vi "TrajectoryDashWrite.vi"(8 "error in (no error)":errorcluster) -> (0 "error out":errorcluster)   [LabVIEW 2023]
uses:
  <vilib>/Rock Robotics/Network Tables/NT Write Boolean.vi
  <vilib>/Rock Robotics/Network Tables/NT Write Numeric Array.vi
  TrajectoryGlobals.vi
  <vilib>/Rock Robotics/Network Tables/NT Write Number.vi
  <vilib>/Rock Robotics/WPI/ThirdParty/JAS_Junk/TrajLib/Trajectory_Library.lvlib
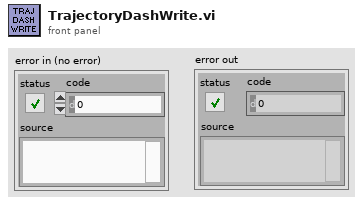
[diagram p1: front panel]
types:
  T1 = typedef "Trajectory_Library.lvlib/POSE2D.ctl" = cluster{"TRANSLATION":T2, "ROTATION":T3}
  T2 = typedef "Trajectory_Library.lvlib/TRANSLATION2D.ctl" = cluster{"X":dbl, "Y":dbl}
  T3 = typedef "Trajectory_Library.lvlib/ROTATION2D.ctl" = cluster{"VALUE":dbl, "COS":dbl, "SIN":dbl}
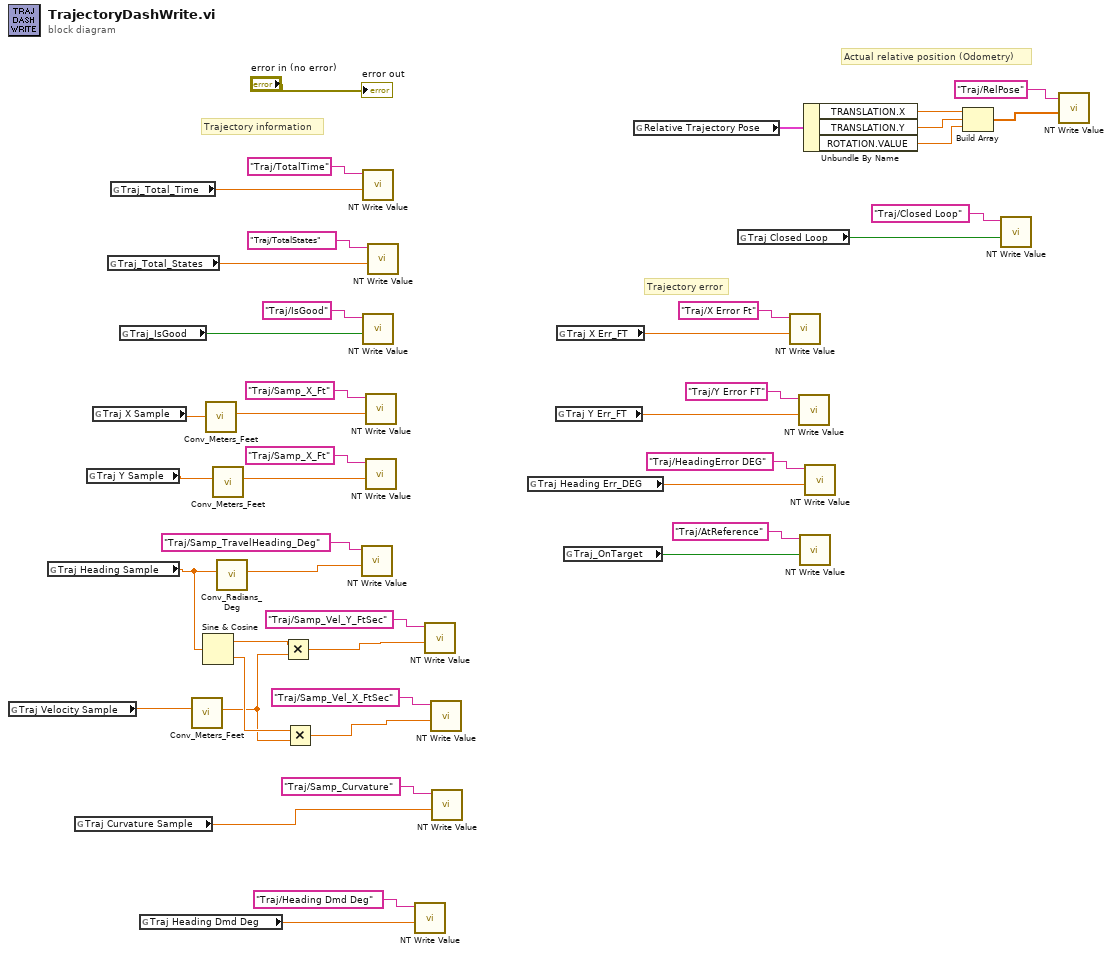
[diagram p0: block diagram]
diagram:
  # "Trajectory information"
  # "Actual relative position (Odometry)"
  # "Trajectory error"
  n1 = global read "TrajectoryGlobals.vi" "Traj Velocity Sample"() -> (w10:dbl)
  n2 = global read "TrajectoryGlobals.vi" "Traj Heading Sample"() -> (w11:dbl)
  n3 = global read "TrajectoryGlobals.vi" "Traj Curvature Sample"() -> (w1:dbl)
  n4 = global read "TrajectoryGlobals.vi" "Traj Y Sample"() -> (w14:dbl)
  n5 = global read "TrajectoryGlobals.vi" "Traj X Sample"() -> (w16:dbl)
  n6 = global read "TrajectoryGlobals.vi" "Traj_Total_States"() -> (w28:dbl)
  n7 = global read "TrajectoryGlobals.vi" "Traj_Total_Time"() -> (w27:dbl)
  n8 = global read "TrajectoryGlobals.vi" "Traj_IsGood"() -> (w29:bool)
  n9 = global read "TrajectoryGlobals.vi" "Traj Heading Dmd Deg"() -> (w25:dbl)
  n10 = call <vilib>:"Conv_Meters_Feet.vi"("Meters"=w10) -> ("Feet"=w5:dbl)  [unwired: 10 in]
  n11 = Sine & Cosine(0:w11) -> (1:w7:dbl, 2:w6:dbl)
  n12 = call <vilib>:"Conv_Meters_Feet.vi"("Meters"=w16) -> ("Feet"=w17:dbl)  [unwired: 10 in]
  n13 = call <vilib>:"Conv_Meters_Feet.vi"("Meters"=w14) -> ("Feet"=w15:dbl)  [unwired: 10 in]
  n14 = call <vilib>:"Conv_Radians_Deg.vi"("Radians"=w11) -> ("Degrees"=w12:dbl)  [unwired: 10 in]
  n15 = Multiply(x=w7, y=w5) -> (x*y=w4:dbl)
  n16 = Multiply(x=w6, y=w5) -> (x*y=w3:dbl)
  n17 = call-poly <vilib>:"NT Write Value.vi"("value"=w12, "name"="Traj/Samp_TravelHeading_Deg" ("Name")) -> ()  [unwired: 9 in, 1 out]
  n18 = call-poly <vilib>:"NT Write Value.vi"("value"=w27, "name"="Traj/TotalTime" ("Name")) -> ()  [unwired: 9 in, 1 out]
  n19 = call-poly <vilib>:"NT Write Value.vi"("value"=w29, "name"="Traj/IsGood" ("Name")) -> ()  [unwired: 9 in, 1 out]
  n20 = call-poly <vilib>:"NT Write Value.vi"("value"=w17, "name"="Traj/Samp_X_Ft" ("Name")) -> ()  [unwired: 9 in, 1 out]
  n21 = call-poly <vilib>:"NT Write Value.vi"("value"=w15, "name"="Traj/Samp_X_Ft" ("Name")) -> ()  [unwired: 9 in, 1 out]
  n22 = call-poly <vilib>:"NT Write Value.vi"("value"=w28, "name"="Traj/TotalStates" ("Name")) -> ()  [unwired: 9 in, 1 out]
  n23 = call-poly <vilib>:"NT Write Value.vi"("value"=w25, "name"="Traj/Heading Dmd Deg" ("Name")) -> ()  [unwired: 9 in, 1 out]
  n24 = call-poly <vilib>:"NT Write Value.vi"("value"=w4, "name"="Traj/Samp_Vel_Y_FtSec" ("Name")) -> ()  [unwired: 9 in, 1 out]
  n25 = call-poly <vilib>:"NT Write Value.vi"("value"=w3, "name"="Traj/Samp_Vel_X_FtSec" ("Name")) -> ()  [unwired: 9 in, 1 out]
  n26 = call-poly <vilib>:"NT Write Value.vi"("value"=w1, "name"="Traj/Samp_Curvature" ("Name")) -> ()  [unwired: 9 in, 1 out]
  n27 = global read "TrajectoryGlobals.vi" "Traj Heading Err_DEG"() -> (w22:dbl)
  n28 = global read "TrajectoryGlobals.vi" "Traj Y Err_FT"() -> (w24:dbl)
  n29 = global read "TrajectoryGlobals.vi" "Traj X Err_FT"() -> (w23:dbl)
  n30 = global read "TrajectoryGlobals.vi" "Traj_OnTarget"() -> (w21:bool)
  n31 = global read "TrajectoryGlobals.vi" "Relative Trajectory Pose"() -> (w20:T1)
  n32 = global read "TrajectoryGlobals.vi" "Traj Closed Loop"() -> (w26:bool)
  n33 = call-poly <vilib>:"NT Write Value.vi"("value"=w23, "name"="Traj/X Error Ft" ("Name")) -> ()  [unwired: 9 in, 1 out]
  n34 = call-poly <vilib>:"NT Write Value.vi"("value"=w24, "name"="Traj/Y Error FT" ("Name")) -> ()  [unwired: 9 in, 1 out]
  n35 = call-poly <vilib>:"NT Write Value.vi"("value"=w21, "name"="Traj/AtReference" ("Name")) -> ()  [unwired: 9 in, 1 out]
  n36 = Unbundle By Name(w20) -> ("TRANSLATION.X"=w39:dbl, "TRANSLATION.Y"=w40:dbl, "ROTATION.VALUE"=w41:dbl)
  n37 = call-poly <vilib>:"NT Write Value.vi"("value"=w22, "name"="Traj/HeadingError DEG" ("Name")) -> ()  [unwired: 9 in, 1 out]
  n38 = Build Array(w39, w40, w41) -> (w37:dbl[])
  n39 = call-poly <vilib>:"NT Write Value.vi"("value"=w26, "name"="Traj/Closed Loop" ("Name")) -> ()  [unwired: 9 in, 1 out]
  n40 = call-poly <vilib>:"NT Write Value.vi"("value"=w37, "name"="Traj/RelPose" ("Name")) -> ()  [unwired: 9 in, 1 out]
  "error out" <- "error in (no error)"
